vi "generate_signal.vi"(8 "error in (no error)":errorcluster, 9 "fault_enabled":bool=TRUE, 10 "duration_s":dbl=1.0 format="%#_13g", 11 "sampling_rate_hz":dbl=1000.0 format="%#_13g") -> (0 "error out":errorcluster, 3 "measured values":dbl[](array[numeric]))   [LabVIEW 2026]
uses:
  <vilib>/Python/Open Venv Python Session.vi
panel:
  out "Waveform Graph":dbl[](graph)
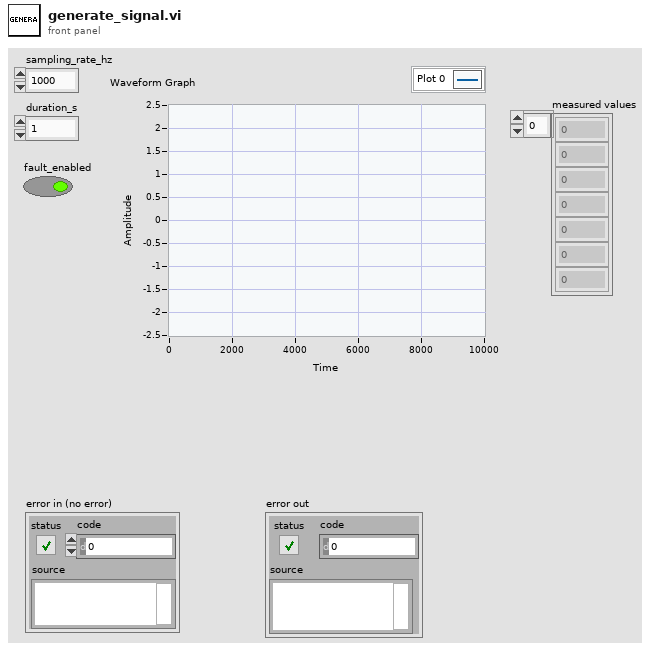
[diagram p1: front panel]
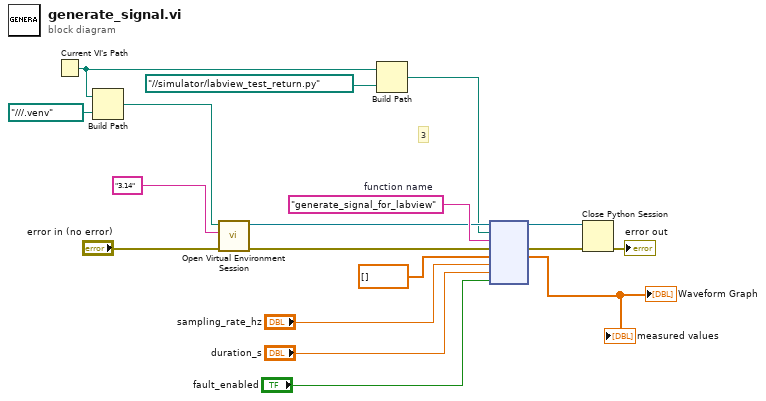
[diagram p0: block diagram]
diagram:
  w18 = "generate_signal_for_labview"  # function name
  # "3"
  n1 = Current VI's Path() -> (path=w7:path)
  n2 = Build Path(base path=w7, name or relative path=path "../../../.venv") -> (appended path=w11:path)
  n3 = call-poly <vilib>:"Open Virtual Environment Session.vi"("error in (no error)"="error in (no error)", "Python version"="3.14", "Env path"=w11) -> ("error out"=w10:errorcluster, "session out"=w8:refnum<k35>)  [unwired: 7 in]
  n4 = Build Path(base path=w7, name or relative path=path "../../simulator/labview_test_return.py") -> (appended path=w2:path)
  n5 = node(w8, w2, w18, w10, dbl[] [] ("b"), "sampling_rate_hz", "duration_s", "fault_enabled") -> (w17:refnum<k35>, w16:errorcluster, →"measured values" →"Waveform Graph":dbl[])  [unwired: 3 in, 2 out]
  n6 = Close Python Session(session in=w17, error in=w16) -> (11:→"error out":errorcluster)
